vi "EJ 4.3.vi"() -> ()   [LabVIEW 2013]
panel:
  in  "Muestras interpol":i32
  in  "Muestras seno":i32
  out "XY Graph":cluster{dbl[], dbl[]}[](graph)
  in  "Frecuencia":dbl
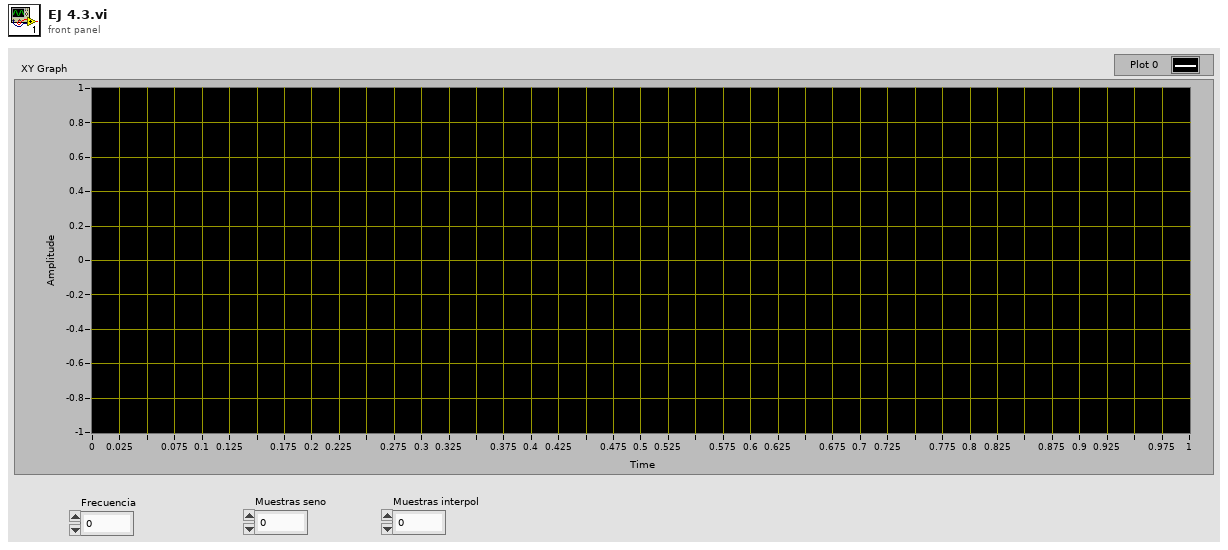
[diagram p1: front panel]
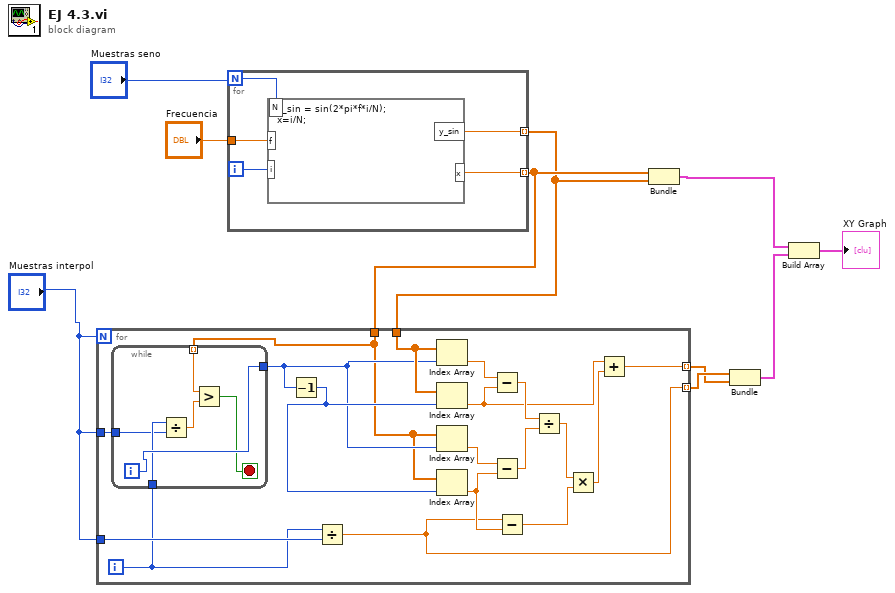
[diagram p0: block diagram]
diagram:
  n1 = for {
    N: "Muestras seno" -> [w15]
    tunnel: "Frecuencia" -> [w14]
    tunnel: [w13] -> w6 mode=indexing
    tunnel: [w12] -> w7 mode=indexing
    i -> [w11]
    n2 = formula code="y_sin = sin(2*pi*f*i/N);\nx=i/N;"("N"=w15, "f"=w14, "i"=w11) -> ("y_sin"=w13:dbl, "x"=w12:dbl)
  }
  n3 = for {
    N: "Muestras interpol" -> [_]
    tunnel: w7 -> [w17]
    tunnel: w6 -> [w31]
    tunnel: "Muestras interpol" -> [w33]
    tunnel: [w23] -> w8 mode=indexing
    tunnel: [w22] -> w9 mode=indexing
    tunnel: "Muestras interpol" -> [w16]
    i -> [w20]
    n4 = while {
      tunnel: w20 -> [w36]
      tunnel: [w38] -> w19
      tunnel: w17 -> [w35] mode=indexing
      tunnel: w16 -> [w34]
      i -> [w38]
      stop <- w37 stop-if-true
      n5 = Divide(x=w36, y=w34) -> (x/y=w39:dbl)
      n6 = Greater?(x=w35, y=w39) -> (0:w37:bool)
    }
    n7 = Decrement(x=w19) -> (x-1=w21:i32)
    n8 = Divide(x=w20, y=w33) -> (x/y=w22:dbl)
    n9 = Index Array(array=w31, index=w19) -> (element=w24:dbl)
    n10 = Index Array(array=w31, index=w21) -> (element=w18:dbl)
    n11 = Index Array(array=w17, index=w19) -> (element=w32:dbl)
    n12 = Index Array(array=w17, index=w21) -> (element=w28:dbl)
    n13 = Subtract(x=w24, y=w18) -> (x-y=w30:dbl)
    n14 = Subtract(x=w32, y=w28) -> (x-y=w29:dbl)
    n15 = Subtract(x=w22, y=w28) -> (x-y=w26:dbl)
    n16 = Divide(x=w30, y=w29) -> (x/y=w27:dbl)
    n17 = Multiply(x=w27, y=w26) -> (x*y=w25:dbl)
    n18 = Add(x=w18, y=w25) -> (x+y=w23:dbl)
  }
  n19 = Bundle(w7, w6) -> (w5:cluster{dbl[], dbl[]})  [unwired: 1 in]
  n20 = Bundle(w9, w8) -> (w4:cluster{dbl[], dbl[]})  [unwired: 1 in]
  n21 = Build Array(w5, w4) -> (→"XY Graph":cluster{dbl[], dbl[]}[])
